vi "close.vi"(8 "error in (no error)":errorcluster, 11 "Analog_Output in":refnum<class "Analog_Output.lvclass">) -> (0 "error out":errorcluster, 3 "Analog_Output out":refnum<class "Analog_Output.lvclass">)   [LabVIEW 2013, in "Analog_Output.lvclass"]
uses:
  Analog_Output.lvclass
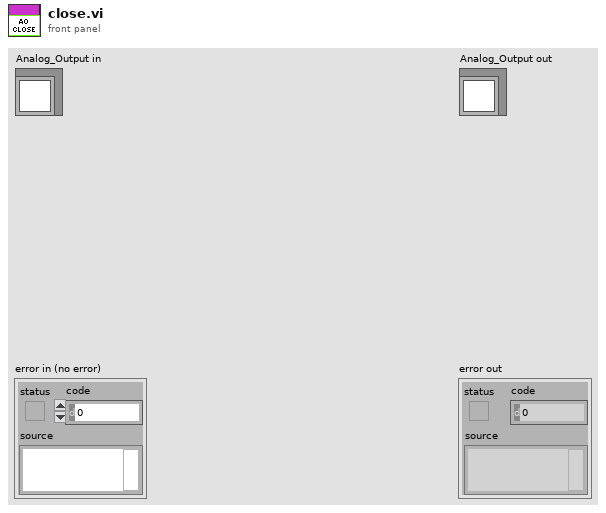
[diagram p1: front panel]
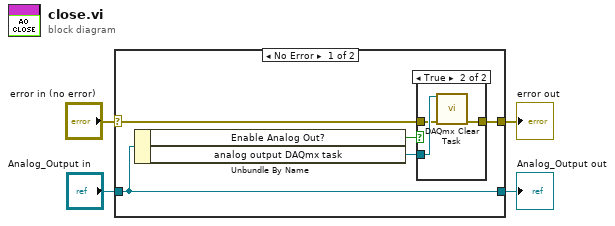
[diagram p0: block diagram]
diagram:
  n1 = case shown="No Error" "error in (no error)" {
    selector: "error in (no error)" -> [w6 w15]
    tunnel: [w5 w15] -> w3
    tunnel: [w9 w14] -> w1
    tunnel: "Analog_Output in" -> [w9 w14]
    frame No Error {
      n2 = Unbundle By Name(w9) -> ("Enable Analog Out?"=w8:bool, "analog output DAQmx task"=w7:refnum<k21>)
      n3 = case shown="True" w8 {
        tunnel: w7 -> [_ w13]
        tunnel: [w10 w12] -> w5
        tunnel: w6 -> [w10 w11]
        frame False {
        }
        frame True {
          n4 = call <vilib>:"DAQmx Clear Task.vi"("task in"=w13, "error in"=w11) -> ("error out"=w12:errorcluster)  [unwired: 13 out]
        }
      }
    }
    frame Error {
    }
  }
  "error out" <- w3
  "Analog_Output out" <- w1
